vi "WPI_AnalogModuleDefaults.vi"() -> (1 "DEFAULT_SAMPLE_RATE":dbl=50000.0, 2 "DEFAULT_OVERSAMPLE_BITS":u8, 3 "DEFAULT_AVERAGE_BITS":u8)   [LabVIEW 2017]
doc: "This software is licensed. Open the labview\\readme\\WPI Robotics Library Open Source License.txt file for more information."
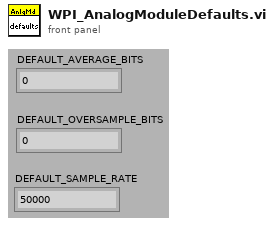
[diagram p1: front panel]
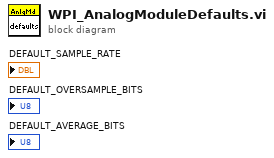
[diagram p0: block diagram]
diagram:
